vi "gotopoints.vi"() -> ()   [LabVIEW 2017]
uses:
  <vilib>/robotics/Navigation/shared/WorldMap/OccupancyGridWorldMap/NI_Robotics_OccupancyGridWorldMap.lvclass
  040-typeDefs/Position.ctl
  <vilib>/myRIO/Common/Instrument Driver Framework/myRIO v1.0/Encoder/typedefs/Encoder Signal Mode.ctl
  <vilib>/myRIO/Instrument Drivers/Onboard IO/Encoder/typedefs/Encoder Reference.ctl
  <vilib>/myRIO/Common/Instrument Driver Framework/Utilities/typedefs/myRIO Generic Hardware Reference.ctl
  <vilib>/myRIO/Common/Instrument Driver Framework/Utilities/typedefs/Hardware Version Enum.ctl
  <vilib>/myRIO/Common/Instrument Driver Framework/Utilities/typedefs/myRIO v1.0 Reference.ctl
  <vilib>/myRIO/Common/Instrument Driver Framework/Utilities/typedefs/Generic FPGA Reference.ctl
  <vilib>/myRIO/Common/Instrument Driver Framework/myRIO v1.0/Encoder/typedefs/Encoder Channels Enum.ctl
  <vilib>/myRIO/Common/Instrument Driver Framework/myRIO v1.0/Encoder/typedefs/Encoder Configuration v1.0.ctl
  <vilib>/userdefined/High Color/nirio_resource_hc.ctl
  <vilib>/myRIO/Common/Instrument Driver Framework/Utilities/vis/Is FPGA Ref Available.vi
  <vilib>/myRIO/Common/Instrument Driver Framework/myRIO v1.0/Encoder/vis/myRIO v1.1 Open Encoder.vi
  <vilib>/myRIO/Instrument Drivers/Onboard IO/Encoder/vis/Read.vi
  <vilib>/myRIO/Common/Instrument Driver Framework/Utilities/vis/Validate Channels.vi
  <vilib>/myRIO/Common/Instrument Driver Framework/myRIO v1.0/Encoder/vis/myRIO v1.0 Reserve Encoder.vi
  <vilib>/myRIO/Common/Instrument Driver Framework/myRIO v1.0/Encoder/vis/myRIO v1.0 Build MUX Configuration Encoder.vi
  <vilib>/myRIO/Common/Instrument Driver Framework/myRIO v1.0/Resource Manager/vis/myRIO v1.0 Reserve Channel List.vi
  <vilib>/myRIO/Common/Instrument Driver Framework/myRIO v1.0/Resource Manager/vis/myRIO v1.0 Create Configuration List.vi
  <vilib>/myRIO/Common/Instrument Driver Framework/myRIO v1.0/Resource Manager/vis/myRIO v1.0 Reserve Channel.vi
  <vilib>/myRIO/Common/Instrument Driver Framework/myRIO v1.0/Resource Manager/vis/myRIO v1.0 Unreserve Channel.vi
  <vilib>/myRIO/Common/Instrument Driver Framework/myRIO v1.0/Resource Manager/vis/myRIO v1.0 Build Mutex Name.vi
  <vilib>/Utility/VariantDataType/GetNumericInfo.vi
  <vilib>/Utility/error.llb/Error Cluster From Error Code.vi
  <vilib>/myRIO/Common/Instrument Driver Framework/myRIO v1.0/myRIO v1.1 Open.vi
  <vilib>/myRIO/Common/Instrument Driver Framework/Utilities/vis/IO Manager.vi
  <vilib>/myRIO/Common/Instrument Driver Framework/Utilities/vis/Configuration Manager.vi
  <vilib>/myRIO/Common/Instrument Driver Framework/myRIO v1.0/Resource Manager/vis/myRIO v1.0 Configure IO.vi
  <vilib>/myRIO/Common/Instrument Driver Framework/myRIO v1.0/myRIO v1.0 Close.vi
  <vilib>/myRIO/Common/Instrument Driver Framework/myRIO v1.0/Encoder/vis/myRIO v1.0 Configure Encoder.vi
  <vilib>/myRIO/Common/Instrument Driver Framework/myRIO v1.0/Encoder/vis/myRIO v1.0 Read Encoder.vi
  <vilib>/addons/control/pid/pid.llb/PID (DBL).vi
  <vilib>/myRIO/Express VI/Onboard IO/Encoder/Encoder Express VI.xnode
  <vilib>/myRIO/Instrument Drivers/Onboard IO/Encoder/vis/myRIO Encoder Open.xnode
  <vilib>/myRIO/Common/Instrument Driver Framework/myRIO v1.0/Encoder/typedefs/Encoder Count Direction Enum.ctl
  <vilib>/addons/control/pid/NI_PID_pid.lvlib
  <vilib>/myRIO/Instrument Drivers/Onboard IO/Encoder/Encoder.lvlib
  <vilib>/Analysis/NI_AALPro.lvlib
panel:
  in  "Robot Relative Position":cluster{"PosX":dbl, "PosY":dbl}
  in  "Boolean 2":bool
  in  "Boolean":bool
  in  "stop 4":bool
  in  "Next Point 2":T1={"X Pos"=250.0, "Y Pos"=190.0, "Bearing"=0.0}
  out "reached":bool=TRUE
  in  "Position":T1
  in  "endPos":cluster{"x":i32, "y":i32}={"x"=6, "y"=3}
  out "path":cluster{"X":i32, "Y":i32}[](array[cluster])=[{"X"=2, "Y"=0}, {"X"=3, "Y"=1}, {"X"=4, "Y"=0}, {"X"=5, "Y"=0}, {"X"=6, "Y"=1}, {"X"=6, "Y"=2}, {"X"=6, "Y"=3}, {"X"=7, "Y"=4}, {"X"=8, "Y"=4}, {"X"=9, "Y"=4}, {"X"=10, "Y"=5}, {"X"=11, "Y"=6}, {"X"=11, "Y"=7}, {"X"=10, "Y"=8}, {"X"=9, "Y"=8}, {"X"=8, "Y"=8}, {"X"=7, "Y"=8}, {"X"=6, "Y"=8}, {"X"=5, "Y"=8}, {"X"=4, "Y"=8}]
  in  "stop 3":bool
  in  "occupancy grid":dbl[][](array[numeric])=[[0.0, 0.0, 0.0, 0.0, 0.0, 0.0, 0.0], [0.0, 0.0, 0.0, 0.0, 0.0, 0.0, 0.0], [0.0, 0.0, 0.0, 0.0, 0.0, 0.0, 0.0], [0.0, 0.0, 0.0, 0.0, 0.0, 0.0, 0.0], [0.0, 15.0, 0.0, 0.0, 0.0, 0.0, 0.0], [0.0, 0.0, 0.0, 0.0, 0.0, 0.0, 0.0], [630.0, 4825.0, 27.0, 0.0, 0.0, 0.0, 0.0]]
  out "XY Graph 3":cluster{i32[], i32[]}(graph)={[300, 400, 500, 600, 600, 600, 700, 800, 900, 1000, 1100, 1100, 1000, 900, 800, 700, 600, 500, 400], [100, 0, 0, 100, 200, 300, 400, 400, 400, 500, 600, 700, 800, 800, 800, 800, 800, 800, 800]}
  out "Pathing Frequency":u32=4294967295
  in  "map reference in 2":refnum<data-value>
  in  "map reference in":refnum<data-value>
  in  "stop 2":bool
  out "output cluster":cluster{"PosX":dbl, "PosY":dbl}={"PosX"=1.0, "PosY"=5.0}
  in  "Resolution":dbl=100.0
  out "Intensity Graph":dbl[][](graph)=[[0.0, 0.0, 0.0, 0.0, 0.0, 0.0, 0.0], [0.0, 0.0, 0.0, 0.0, 0.0, 0.0, 0.0], [0.0, 0.0, 0.0, 0.0, 0.0, 0.0, 0.0], [0.0, 0.0, 0.0, 0.0, 0.0, 0.0, 0.0], [0.0, 15.0, 0.0, 0.0, 0.0, 0.0, 0.0], [0.0, 0.0, 0.0, 0.0, 0.0, 0.0, 0.0], [630.0, 4825.0, 27.0, 0.0, 0.0, 0.0, 0.0]]
  out "Frequency":u32=10
  out "XY Graph 2":cluster{dbl[], dbl[]}(graph)
  out "Setpoint B":dbl(slide)=2.4299999999999997 scale=-10.0..10.0
  out "Setpoint A":dbl(slide)=0.42999999999999994 scale=-10.0..10.0
  out "PID B":T2(graph)
  out "PID A":T2(graph)
  out "OUTPUT A":dbl(slide) scale=-10.0..10.0
  out "OUTPUT B":dbl(slide) scale=-10.0..10.0
  in  "stop":bool
  in  "PID gains":T3={"proportional gain (Kc)"=0.05, "integral time (Ti, min)"=0.05, "derivative time (Td, min)"=0.0} {"derivative time (Td, min)" format="%.3f"; "integral time (Ti, min)" format="%.3f"; "proportional gain (Kc)" format="%.3f"}
  out "XY Graph":cluster{"X":dbl, "Y":dbl}[](graph)=[{"X"=540.9440365841652, "Y"=149.8526832016017}, {"X"=540.9440365841652, "Y"=149.8526832016017}]
  out "PID Angle":cluster{"Bearing":dbl, dbl}(graph)={"Bearing"=6886.263626973743, 6998.426769231998}
  out "X, Y, BEARING 2":cluster{dbl, dbl, dbl}={540.9440365841652, 149.8526832016017, 6998.426769231998}
  in  "threshold":dbl=100.0
  in  "Max Speed":dbl=2.0
  in  "Min Speed":dbl=1.0
  in  "Initial X, Y, BEARING":cluster{dbl, dbl, dbl}={10.0, 350.0, 0.0}
  out "Final X, Y, BEARING":cluster{dbl, dbl, dbl}={245.38756896666968, 124.45046063453532, -26.464846153846153}
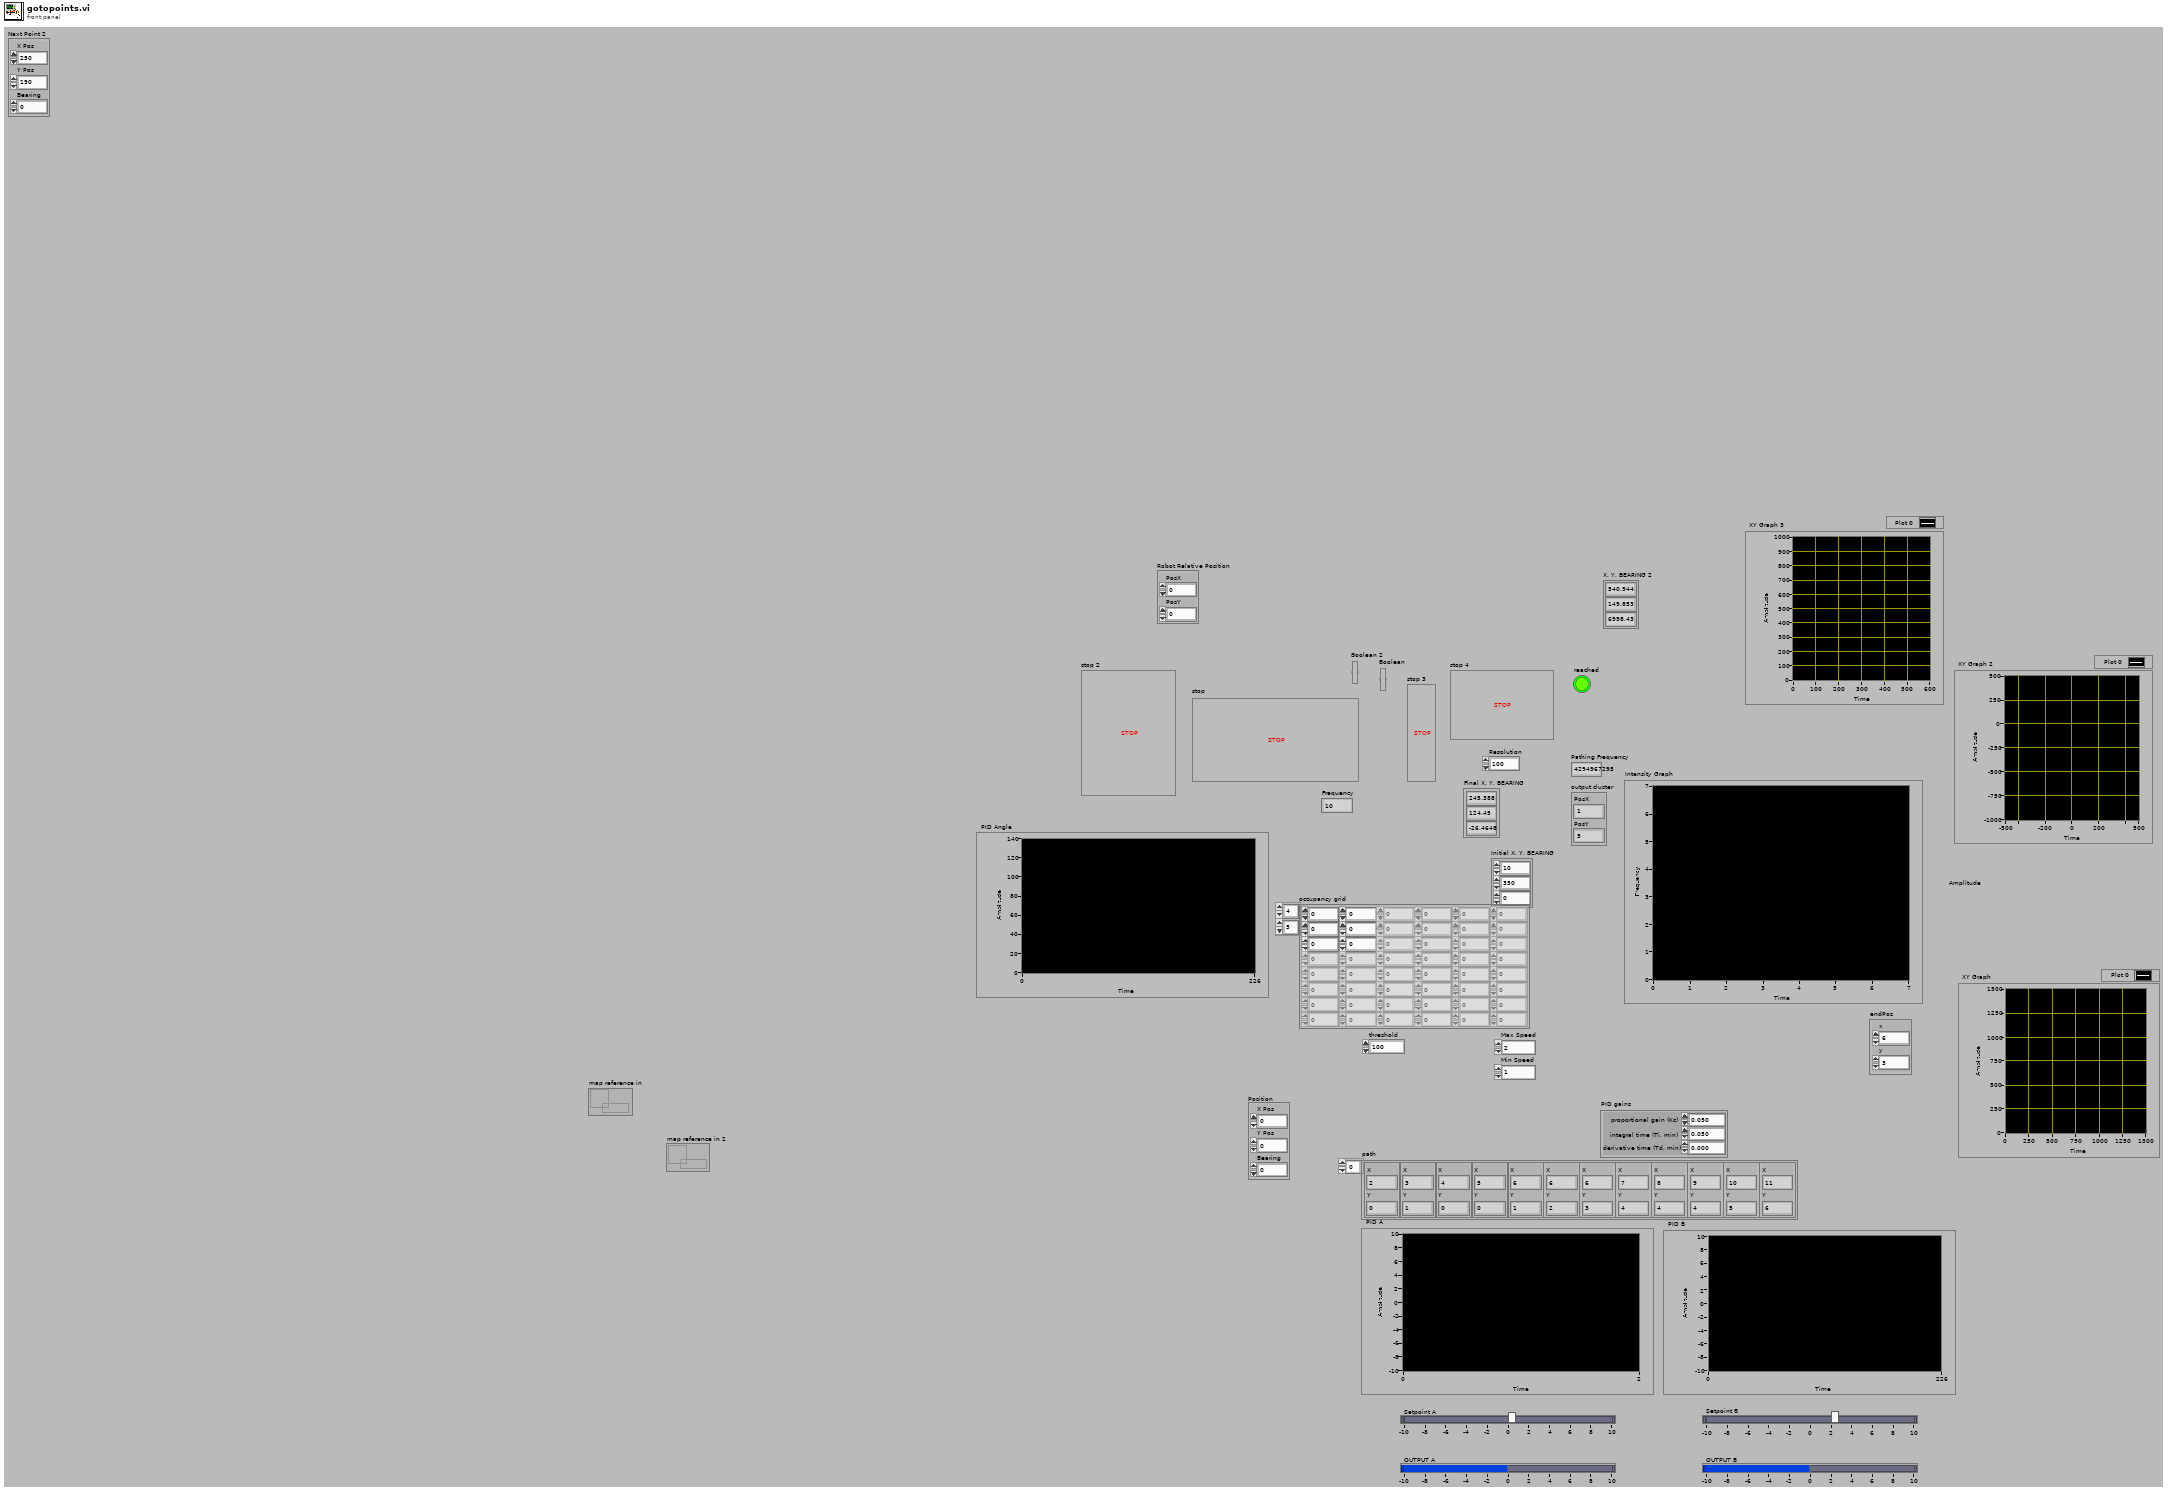
[diagram p1: front panel]
types:
  T1 = typedef "Position.ctl" = cluster{"X Pos":dbl, "Y Pos":dbl, "Bearing":dbl}
  T2 = cluster{"Setpoint":dbl, "output":dbl, "dx/dt":dbl}
  T3 = cluster{"proportional gain (Kc)":dbl, "integral time (Ti, min)":dbl, "derivative time (Td, min)":dbl}
  T4 = typedef "Encoder.lvlib/Encoder Reference.ctl" = cluster{"myRIO Reference":T5, "Encoder Channels Enum":T9}
  T5 = typedef "myRIO Generic Hardware Reference.ctl" = cluster{"myRIO Model":T6, "myRIO Hardware Reference":T7}
  T6 = typedef "Hardware Version Enum.ctl" = enum16{"Unknown", "myRIO-1900", "myRIO-1950", "roboRIO", "NI ELVIS RIO CM"}
  T7 = typedef "myRIO v1.0 Reference.ctl" = cluster{"Generic FPGA Reference":T8, "Allow multiple opens":bool}
  T8 = typedef "Generic FPGA Reference.ctl" = refnum<k20>
  T9 = typedef "Encoder Channels Enum.ctl" = enum16{"Not Connected", "C/ENC0", "C/ENC1", "A/ENC", "B/ENC", "DIO/ENC0", "DIO/ENC1", "DIO/ENC2", "DIO/ENC3", "DIO/ENC4"}
  T10 = typedef "Encoder Signal Mode.ctl" = enum16{"Quadrature phase signal", "Step and direction signal"}
  T11 = typedef "nirio_resource_hc.ctl" = tag
  T12 = typedef "LidarPoint.ctl" = cluster{"X":dbl, "Y":dbl}
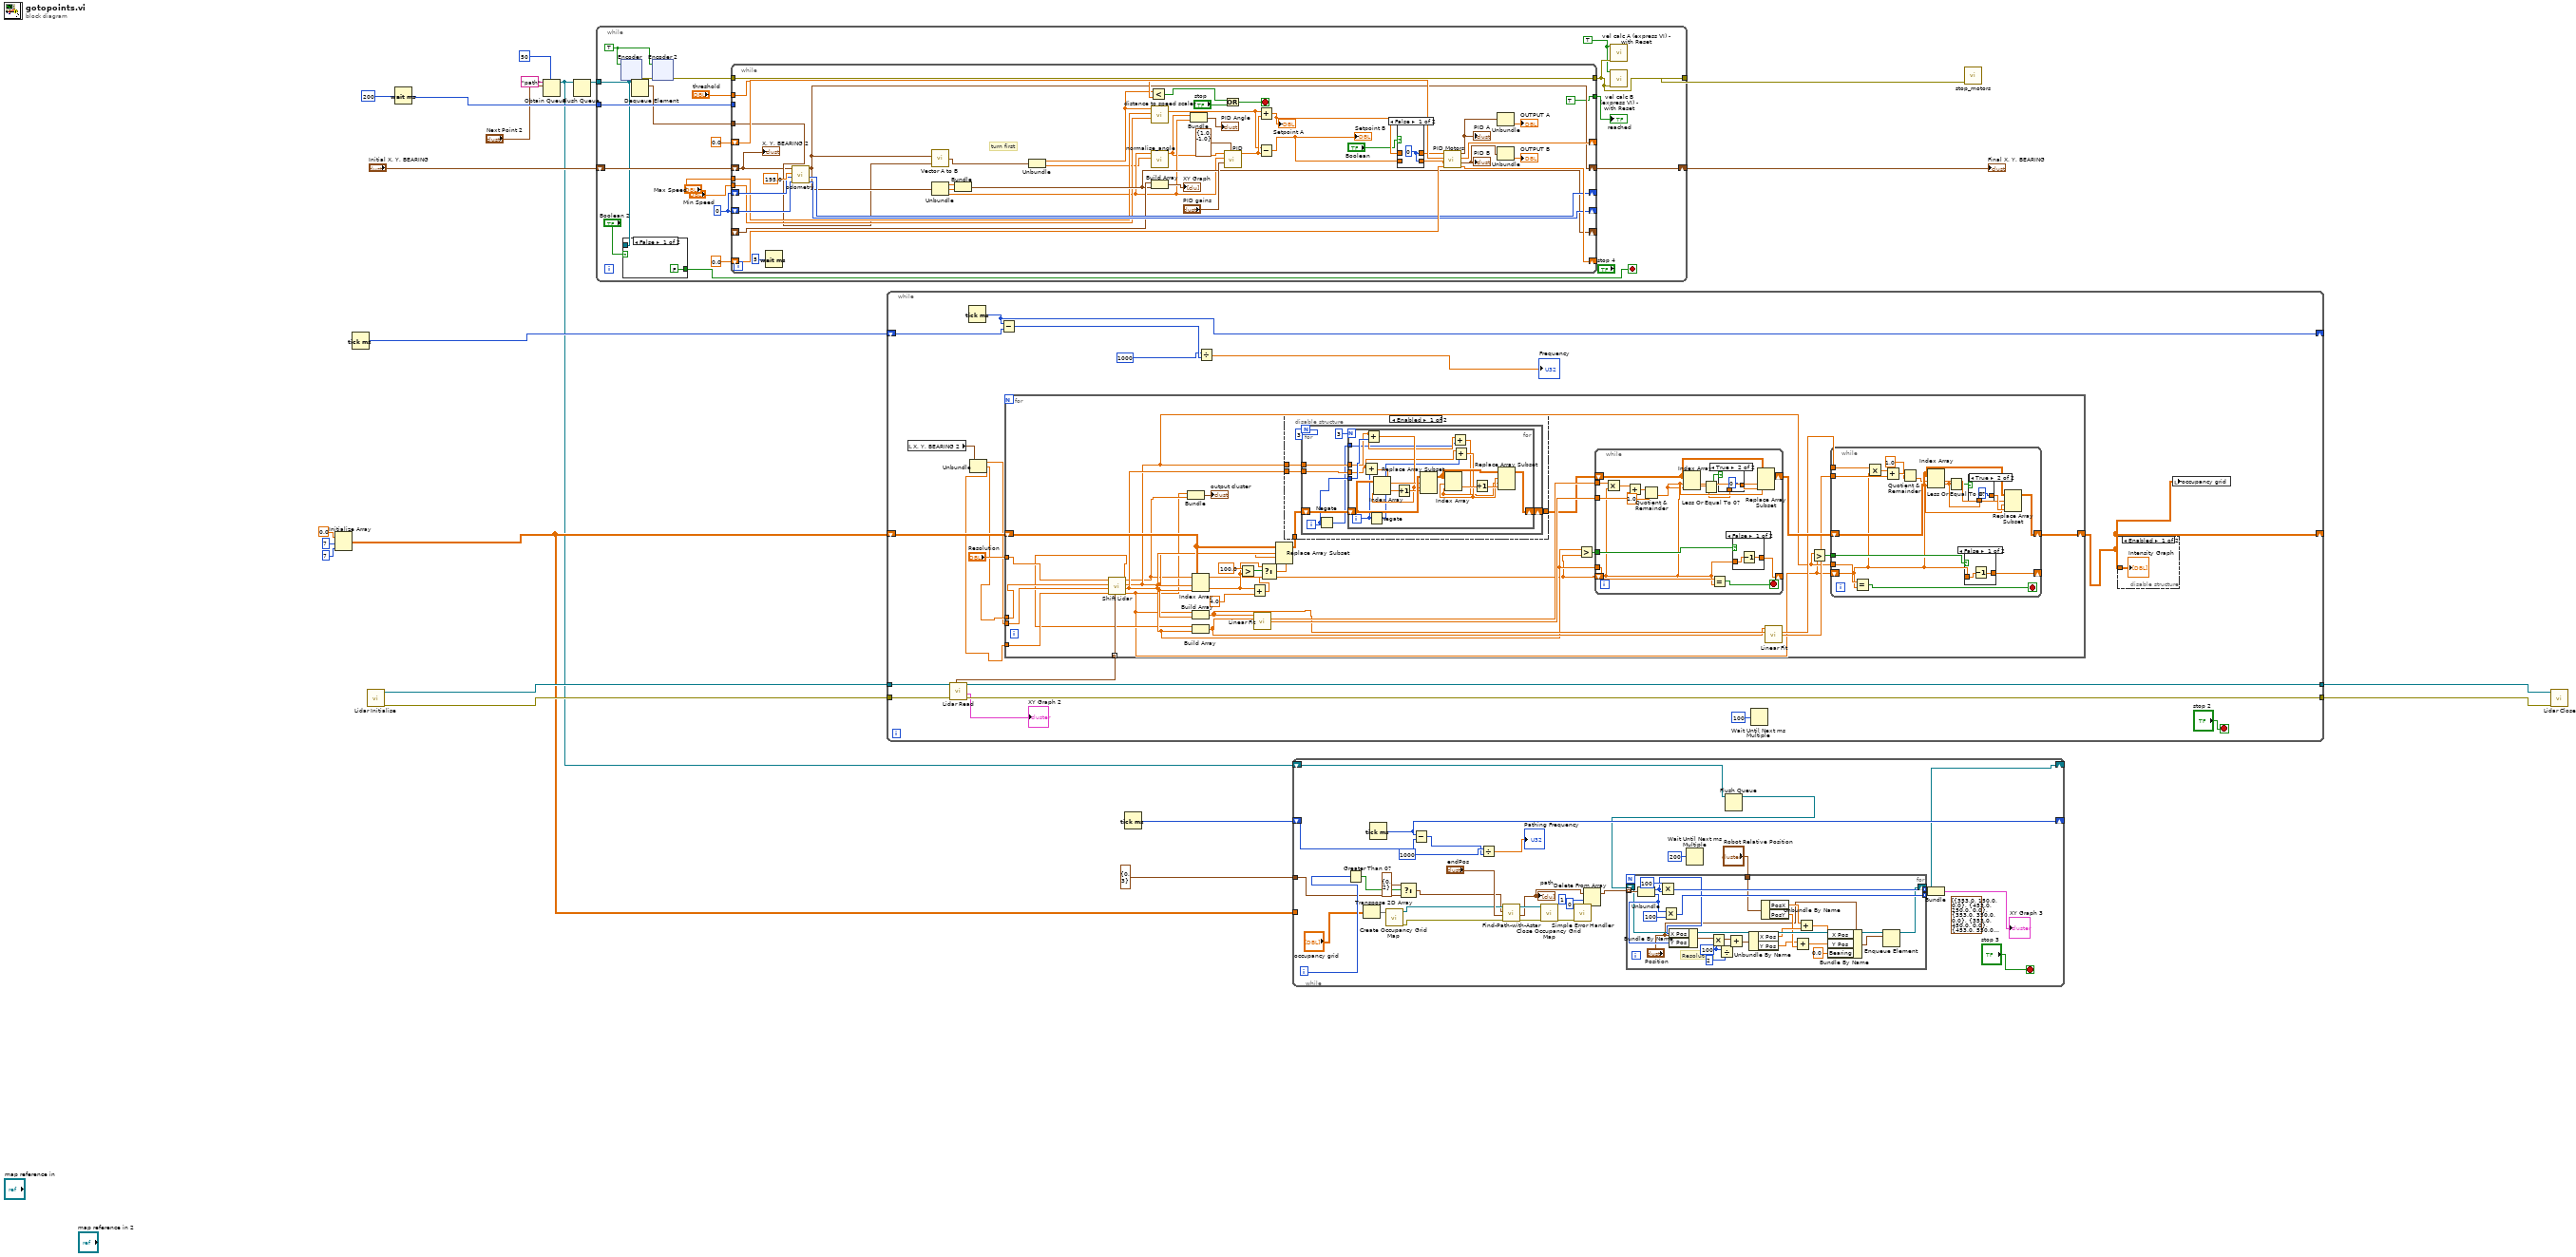
[diagram p0: block diagram]
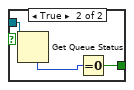
[diagram p2: hidden frame]
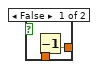
[diagram p6: hidden frame]
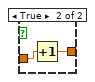
[diagram p7: hidden frame]
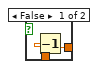
[diagram p8: hidden frame]
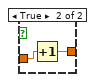
[diagram p9: hidden frame]
diagram:
  n1 = Initialize Array(0.0 ("element"), 7 ("dimension size"), 7 ("dimension size")) -> (w4:dbl[][])
  n2 = Tick Count (ms)() -> (millisecond timer value=w9:u32)
  n3 = call "Lidar Initialise.vi"() -> ("error out"=w15:errorcluster, "VISA resource name out"=w16:refnum<visa-resource-name>)  [unwired: 10 in]
  n4 = Wait (ms)(milliseconds to wait=u32 200) -> (millisecond timer value=w17:u32)
  n5 = Obtain Queue(max queue size (-1, unlimited)=50, name (unnamed)="path", element data type="Next Point 2") -> (queue out=w2:refnum<queue>)  [unwired: 2 in, 2 out]
  n6 = Flush Queue(queue=w2) -> (queue out=w1:refnum<queue>)  [unwired: 1 in, 2 out]
  n7 = while {
    tunnel: [w39] -> w20
    tunnel: w17 -> [w38]
    tunnel: w1 -> [w24]
    shift-right: [w40] -> w21
    shift-left: "Initial X, Y, BEARING" -> [w25]
    stop <- w23 stop-if-true
    w27 = TRUE ("Reinitialise")
    w30 = TRUE
    w34 = 0 ("ENCA OUT")
    n8 = xnode "Encoder"("Reset Counter"=w30) -> ("error out"=w31:errorcluster)  [unwired: 1 in, 3 out]
    n9 = case shown="False" "Boolean 2" {
      tunnel: w24 -> [_ w44]
      tunnel: [FALSE w42] -> w23
      frame False {
      }
      frame True {
        n10 = Get Queue Status(queue=w44) -> (# elements in queue=w43:i32)  [unwired: 2 in, 7 out]
        n11 = Equal To 0?(x=w43) -> (x = 0?=w42:bool)
      }
    }
    n12 = Dequeue Element(queue=w24) -> (element=w28:T1)  [unwired: 2 in, 3 out]
    n13 = xnode "Encoder 2"("error in (no error)"=w31, "Reset Counter"=w30) -> ("error out"=w29:errorcluster)  [unwired: 3 out]
    n14 = while {
      tunnel: w29 -> [w175]
      shift-right: [w177] -> _
      shift-left: 0.0 ("output A") -> [w178]
      shift-right: [w180] -> _
      shift-left: 0.0 ("output B") -> [w179]
      tunnel: [w175] -> w39
      tunnel: "threshold" -> [w165]
      shift-right: [w161] -> _
      shift-left: w34 -> [w163]
      shift-right: [w160] -> _
      shift-left: w34 -> [w162]
      shift-right: [w159] -> w40
      shift-left: w25 -> [w142]
      shift-right: [w155] -> _
      shift-left: _ -> [w156]
      tunnel: "Max Speed" -> [w150]
      tunnel: "Min Speed" -> [w149]
      tunnel: w38 -> [_]
      tunnel: [TRUE ("Reinitialise")] -> w26
      tunnel: w28 -> [w143]
      stop <- w166 stop-if-true
      # "turn first"
      n15 = Wait (ms)(milliseconds to wait=5 ("ENCB OUT")) -> ()  [unwired: 1 out]
      n16 = call "odometry.vi"("ENCB in"=w162, "ENCA in"=w163, "wheelbase"=195.0, "Position"=w142) -> ("ENCB OUT"=w160:i32, "ENCA OUT"=w161:i32, "X, Y, BEARING"=w159:cluster{dbl, dbl, dbl})  [unwired: 4 in]
      n17 = call "Vector A to B.vi"("Destination"=w143, "Current"=w159) -> ("vector"=w168:cluster{dbl, "Bearing":dbl})
      n18 = Unbundle(w159) -> (w157:dbl, w158:dbl, w147:dbl)
      n19 = Bundle(w157, w158) -> (w155:cluster{dbl, dbl})  [unwired: 1 in]
      n20 = Unbundle(w168) -> (w151:dbl, "Bearing"=w146:dbl)
      n21 = Less?(x=w151, y=w165) -> (x < y?=w164:bool)
      n22 = call "distance to speed scaler.vi"("Min Speed"=w149, "Max Speed"=w150, "Distance (mm)"=w151) -> ("Speed (0..10)"=w152:dbl)  [unwired: 2 in]
      n23 = call "normalise_angle.vi"("target -180 .. 180"=w146, "current"=w147) -> ("travel_direction"=w145:dbl)  [unwired: 9 in]
      n24 = Build Array(w156, w155) -> (→"XY Graph":cluster{dbl, dbl}[])
      n25 = Bundle("travel_direction"=w145, w147) -> (→"PID Angle":cluster{"travel_direction":dbl, dbl})  [unwired: 1 in]
      n26 = Or(x=w164, y="stop") -> (x .or. y?=w166:bool)
      n27 = call-poly <vilib>:"PID.vi"("output range"=cluster{"output high":dbl, "output low":dbl} {"output high"=1.0, "output low"=-1.0}, "PID gains"="PID gains", "process variable"=w147, "setpoint"=w145) -> ("output"=w170:dbl)  [unwired: 6 in, 1 out]
      n28 = Add(x=w152, y=w170) -> (x+y=w140:dbl)
      "Setpoint A" <- w140
      n29 = Subtract(x=w152, y=w170) -> (x-y=w138:dbl)
      "Setpoint B" <- w138
      n30 = case shown="False" "Boolean" {
        tunnel: [w182 w184] -> w141
        tunnel: w140 -> [_ w184]
        tunnel: [w182 w183] -> w139
        tunnel: w138 -> [_ w183]
        frame False {
          w182 = 0
        }
        frame True {
        }
      }
      n31 = call "PID Motors.vi"("input B"=w179, "Speed B"=w139, "input A"=w178, "Speed A"=w141) -> ("output B"=w180:dbl, "Speed B0"=w173:T2, "output A"=w177:dbl, "Speed A0"=w174:T2)
      "PID B" <- w173
      "PID A" <- w174
      n32 = Unbundle(w174) -> ("dx/dt"=→"OUTPUT A":dbl)  [unwired: 2 out]
      n33 = Unbundle(w173) -> ("dx/dt"=→"OUTPUT B":dbl)  [unwired: 2 out]
      "X, Y, BEARING 2" <- w142
    }
    "reached" <- w26
    n34 = call "vel calc A (express VI) - with Reset.vi"("error in"=w39, "Reinitialise"=w27) -> ()  [unwired: 5 in, 5 out]
    n35 = call "vel calc B (express VI) - with Reset.vi"("error in"=w39, "Reinitialise"=w27) -> ()  [unwired: 5 in, 5 out]
  }
  "Final X, Y, BEARING" <- w21
  n36 = while {
    tunnel: w16 -> [w204]
    tunnel: w15 -> [w203]
    tunnel: [w202] -> w14
    tunnel: [w201] -> w13
    shift-right: [w191] -> _
    shift-left: w4 -> [w198]
    shift-right: [w195] -> _
    shift-left: w9 -> [w197]
    stop <- "stop 2" stop-if-true
    n37 = local read "X, Y, BEARING 2"() -> (w188:cluster{dbl, dbl, dbl})
    n38 = call "Lidar Read.vi"("error in (no error)"=w203, "VISA resource name"=w204) -> ("error out"=w201:errorcluster, "Visual Out"=→"XY Graph 2":cluster{dbl[], dbl[]}, "VISA resource name out"=w202:refnum<visa-resource-name>, "XYflipped"=w192:T12[])  [unwired: 2 in, 3 out]
    n39 = Tick Count (ms)() -> (millisecond timer value=w195:u32)
    n40 = Unbundle(w188) -> (w186:dbl, w187:dbl, w185:dbl)
    n41 = Subtract(x=w195, y=w197) -> (x-y=w194:u32)
    n42 = for {
      tunnel: w187 -> [w232]
      tunnel: w186 -> [w227]
      tunnel: "Resolution" -> [w234]
      tunnel: w192 -> [w233] mode=indexing
      shift-right: [w212] -> w191
      shift-left: w198 -> [w231]
      tunnel: w185 -> [w211]
      n43 = call "Shift Lidar.vi"("XY"=w233, "Angle"=w211, "X position"=w227, "Y position"=w232, "Resolution"=w234) -> ("PosY"=w208:dbl, "Shifted X"=w214:dbl, "Shifted Y"=w213:dbl, "PosX"=w209:dbl)  [unwired: 3 in]
      n44 = Bundle("PosY"=w208, "PosX"=w209) -> (→"output cluster":cluster{"PosY":dbl, "PosX":dbl})  [unwired: 1 in]
      n45 = Index Array(array=w231, index (row)=w214, index (col)=w213) -> (element=w215:dbl)
      n46 = Build Array(w208, w213) -> (w223:dbl[])
      n47 = Build Array(w209, w214) -> (w222:dbl[])
      n48 = Greater?(x=100.0, y=w215) -> (0:w218:bool)
      n49 = Add(x=w215, y=4.0) -> (x+y=w216:dbl)
      n50 = call <vilib>:"Linear Fit.vi"("Y"=w223, "X"=w222) -> ("slope"=w230:dbl, "intercept"=w229:dbl)  [unwired: 9 in, 3 out]
      n51 = Select(t=w215, s=w218, f=w216) -> (s? t:f=w219:dbl)
      n52 = Replace Array Subset(array=w231, new element=w219, index (row)=w214, index (col)=w213) -> (w207:dbl[][])
      n53 = disable-structure shown="Enabled" {
        disable-tunnel: w214 -> [w238 _]
        disable-tunnel: w213 -> [w237 _]
        disable-tunnel: w207 -> [w236 _]
        disable-tunnel: [w235 _] -> w206
        frame Enabled {
          n54 = for {
            N: 3 -> [_]
            tunnel: w238 -> [w244]
            tunnel: w237 -> [w242]
            shift-right: [w245] -> w235
            shift-left: w236 -> [w246]
            i -> [w241]
            n55 = Negate(x=w241) -> (-x=w240:i32)
            n56 = for {
              N: 3 -> [_]
              tunnel: w244 -> [w251]
              tunnel: w242 -> [w252]
              tunnel: w241 -> [w256]
              tunnel: w240 -> [w250]
              shift-right: [w259] -> w245
              shift-left: w246 -> [w261]
              i -> [w257]
              n57 = Add(x=w251, y=w257) -> (x+y=w254:dbl)
              n58 = Add(x=w252, y=w256) -> (x+y=w253:dbl)
              n59 = Negate(x=w257) -> (-x=w249:i32)
              n60 = Index Array(array=w261, index (row)=w254, index (col)=w253) -> (element=w263:dbl)
              n61 = Increment(x=w263) -> (x+1=w255:dbl)
              n62 = Replace Array Subset(array=w261, new element=w255, index (row)=w254, index (col)=w253) -> (w260:dbl[][])
              n63 = Add(x=w252, y=w250) -> (x+y=w247:dbl)
              n64 = Add(x=w251, y=w249) -> (x+y=w248:dbl)
              n65 = Index Array(array=w260, index (row)=w248, index (col)=w247) -> (element=w262:dbl)
              n66 = Increment(x=w262) -> (x+1=w258:dbl)
              n67 = Replace Array Subset(array=w260, new element=w258, index (row)=w248, index (col)=w247) -> (w259:dbl[][])
            }
          }
        }
        frame Disabled {
        }
      }
      n68 = Greater?(x=w214, y=w209) -> (0:w228:bool)
      n69 = while {
        tunnel: w214 -> [w301]
        shift-right: [w299] -> _
        shift-left: w209 -> [w294]
        tunnel: w230 -> [w298]
        tunnel: w229 -> [w296]
        tunnel: w228 -> [w300]
        shift-right: [w293] -> w225
        shift-left: w206 -> [w295]
        stop <- w302 stop-if-true
        n70 = Multiply(x=w298, y=w294) -> (x*y=w297:dbl)
        n71 = Add(x=w297, y=w296) -> (x+y=w290:dbl)
        n72 = Quotient & Remainder(x=w290, y=1.0) -> (floor(x/y)=w288:dbl)  [unwired: 1 out]
        n73 = Index Array(array=w295, index (row)=w294, index (col)=w288) -> (element=w291:dbl)
        n74 = Less Or Equal To 0?(x=w291) -> (x <= 0?=w287:bool)
        n75 = Equal?(x=w301, y=w294) -> (x = y?=w302:bool)
        n76 = case shown="True" w287 {
          tunnel: [w304 0] -> w292
          tunnel: w291 -> [w303 _]
          frame False {
            n77 = Decrement(x=w303) -> (x-1=w304:dbl)
          }
          frame True {
          }
        }
        n78 = case shown="False" w300 {
          tunnel: w294 -> [w306 w309]
          tunnel: [w307 w308] -> w299
          frame False {
            n79 = Decrement(x=w306) -> (x-1=w307:dbl)
          }
          frame True {
            n80 = Increment(x=w309) -> (x+1=w308:dbl)
          }
        }
        n81 = Replace Array Subset(array=w295, new element=w292, index (row)=w294, index (col)=w288) -> (w293:dbl[][])
      }
      n82 = call <vilib>:"Linear Fit.vi"("Y"=w222, "X"=w223) -> ("slope"=w221:dbl, "intercept"=w220:dbl)  [unwired: 9 in, 3 out]
      n83 = Greater?(x=w213, y=w208) -> (0:w224:bool)
      n84 = while {
        shift-right: [w269] -> w212
        shift-left: w225 -> [w268]
        shift-right: [w276] -> _
        shift-left: w208 -> [w266]
        tunnel: w213 -> [w278]
        tunnel: w224 -> [w277]
        tunnel: w221 -> [w275]
        tunnel: w220 -> [w273]
        stop <- w279 stop-if-true
        n85 = Equal?(x=w278, y=w266) -> (x = y?=w279:bool)
        n86 = Multiply(x=w275, y=w266) -> (x*y=w274:dbl)
        n87 = Add(x=w274, y=w273) -> (x+y=w272:dbl)
        n88 = Quotient & Remainder(x=w272, y=1.0) -> (floor(x/y)=w265:dbl)  [unwired: 1 out]
        n89 = Index Array(array=w268, index (row)=w265, index (col)=w266) -> (element=w270:dbl)
        n90 = Less Or Equal To 0?(x=w270) -> (x <= 0?=w264:bool)
        n91 = case shown="False" w277 {
          tunnel: w266 -> [w283 w286]
          tunnel: [w284 w285] -> w276
          frame False {
            n92 = Decrement(x=w283) -> (x-1=w284:dbl)
          }
          frame True {
            n93 = Increment(x=w286) -> (x+1=w285:dbl)
          }
        }
        n94 = case shown="True" w264 {
          tunnel: [w281 0] -> w267
          tunnel: w270 -> [w280 _]
          frame False {
            n95 = Decrement(x=w280) -> (x-1=w281:dbl)
          }
          frame True {
          }
        }
        n96 = Replace Array Subset(array=w268, new element=w267, index (row)=w265, index (col)=w266) -> (w269:dbl[][])
      }
    }
    n97 = Divide(x=u32 1000 ("y"), y=w194) -> (x/y=→"Frequency":dbl)
    n98 = Wait Until Next ms Multiple(millisecond multiple=u32 100) -> ()  [unwired: 1 out]
    n99 = disable-structure shown="Enabled" {
      disable-tunnel: w191 -> [w205 _]
      frame Enabled {
        "Intensity Graph" <- w205
      }
      frame Disabled {
      }
    }
    n100 = local write "occupancy grid"(w191) -> ()
  }
  n101 = Tick Count (ms)() -> (millisecond timer value=w8:u32)
  n102 = while {
    shift-right: [w329] -> _
    shift-left: w8 -> [w330]
    tunnel: cluster{"x":i32, "y":i32} {"x"=0, "y"=3} ("endPos") -> [w318]
    shift-right: [w320] -> _
    shift-left: w2 -> [w321]
    tunnel: w4 -> [_]
    i -> [w325]
    stop <- "stop 3" stop-if-true
    (unwired) T1[] [{"X Pos"=353.0, "Y Pos"=150.0, "Bearing"=0.0}, {"X Pos"=453.0, "Y Pos"=250.0, "Bearing"=0.0}, {"X Pos"=353.0, "Y Pos"=350.0, "Bearing"=0.0}, {"X Pos"=353.0, "Y Pos"=450.0, "Bearing"=0.0}, {"X Pos"=453.0, "Y Pos"=550.0, "Bearing"=0.0}, {"X Pos"=453.0, "Y Pos"=650.0, "Bearing"=0.0}, {"X Pos"=353.0, "Y Pos"=650.0, "Bearing"=0.0}] ("Array")
    n103 = Greater Than 0?(x=w325) -> (x > 0?=w319:bool)
    n104 = Transpose 2D Array(2D array="occupancy grid") -> (transposed array=w331:dbl[][])
    n105 = Tick Count (ms)() -> (millisecond timer value=w329:u32)
    n106 = call <vilib>:"Create Occupancy Grid Map.vi"("occupancy grid"=w331) -> ("error out"=w335:errorcluster, "map reference out"=w336:refnum<data-value>)  [unwired: 9 in]
    n107 = Select(t=cluster{"x":i32, "y":i32} {"x"=0, "y"=2}, s=w319, f=w318) -> (s? t:f=w317:cluster{"x":i32, "y":i32})
    n108 = Subtract(x=w329, y=w330) -> (x-y=w327:u32)
    n109 = Divide(x=u32 1000 ("y"), y=w327) -> (x/y=→"Pathing Frequency":dbl)
    n110 = call "Find-Path-with-Astar.vi"("error in (no error)"=w335, "goal node"="endPos", "start node"=w317, "map reference in"=w336) -> ("error out"=w339:errorcluster, "Array"=w314:cluster{"X":i32, "Y":i32}[], "map reference out"=w340:refnum<data-value>)  [unwired: 5 in]
    "path" <- w314
    n111 = call <vilib>:"Close Occupancy Grid Map.vi"("error in (no error)"=w339, "map reference in"=w340) -> ("error out"=w338:errorcluster)  [unwired: 9 in]
    n112 = call <vilib>:"Simple Error Handler.vi"("error in (no error)"=w338) -> ()  [unwired: 4 in, 5 out]
    n113 = Delete From Array(array=w314, length=1, index=0) -> (array with subset deleted=w315:cluster{"X":i32, "Y":i32}[])  [unwired: 1 out]
    n114 = Wait Until Next ms Multiple(millisecond multiple=u32 200) -> ()  [unwired: 1 out]
    n115 = Flush Queue(queue=w321) -> (queue out=w322:refnum<queue>)  [unwired: 1 in, 2 out]
    n116 = for {
      tunnel: w315 -> [w365] mode=indexing
      tunnel: [w362] -> w333 mode=indexing
      tunnel: [w364] -> w332 mode=indexing
      shift-right: [w356] -> w320
      shift-left: w322 -> [w357]
      tunnel: "Robot Relative Position" -> [w341]
      w354 = 100
      # "Resolution"
      n117 = Unbundle(w365) -> ("X"=w359:i32, "Y"=w358:i32)
      n118 = Multiply(x=100, y=w359) -> (x*y=w362:i32)
      n119 = Multiply(x=w358, y=100) -> (x*y=w364:i32)
      n120 = Bundle By Name(cluster="Position", "X Pos"=w359, "Y Pos"=w358) -> (w360:T1)
      n121 = Multiply(x=w360, y=w354) -> (x*y=w355:T1)
      n122 = Divide(x=w354, y=2) -> (x/y=w353:dbl)
      n123 = Add(x=w355, y=w353) -> (x+y=w351:T1)
      n124 = Unbundle By Name(w351) -> ("X Pos"=w349:dbl, "Y Pos"=w347:dbl)
      n125 = Unbundle By Name(w341) -> ("PosX"=w350:dbl, "PosY"=w348:dbl)
      n126 = Add(x=w347, y=w348) -> (x+y=w345:dbl)
      n127 = Add(x=w350, y=w349) -> (x+y=w346:dbl)
      n128 = Bundle By Name(cluster="Position", "X Pos"=w346, "Y Pos"=w345, "Bearing"=0.0) -> (w342:T1)
      n129 = Enqueue Element(queue=w357, element=w342) -> (queue out=w356:refnum<queue>)  [unwired: 2 in, 2 out]
    }
    n130 = Bundle(w333, w332) -> (→"XY Graph 3":cluster{i32[], i32[]})  [unwired: 1 in]
  }
  n131 = call "stop_motors.vi"("error in (no error)"=w20) -> ()  [unwired: 4 in, 1 out]
  n132 = call "Lidar Close.vi"("error in (no error)"=w13, "VISA resource name"=w14) -> ()  [unwired: 9 in, 1 out]
